vi "DigitalToString.vi"(2 "D3":bool, 3 "D2":bool, 4 "D1":bool) -> (0 "Numeric":dbl, 1 "String":string)   [LabVIEW 2014]
panel:
  out "Led 3":bool
  out "Led 2":bool
  out "Led 1":bool
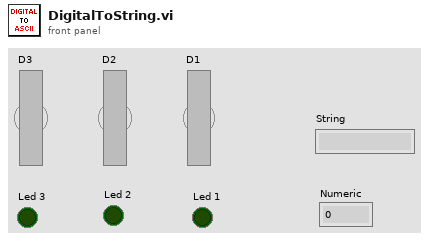
[diagram p1: front panel]
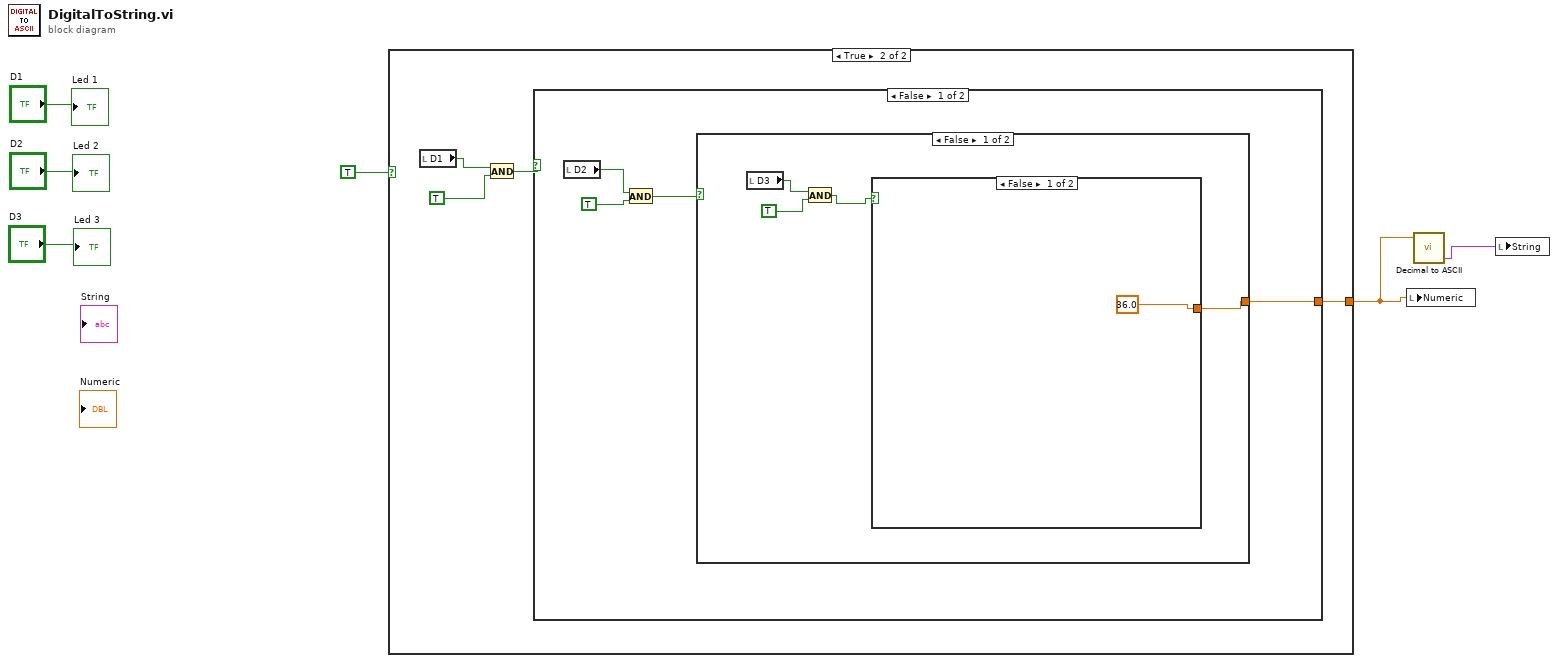
[diagram p0: block diagram]
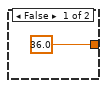
[diagram p2: hidden frame]
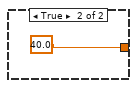
[diagram p3: hidden frame]
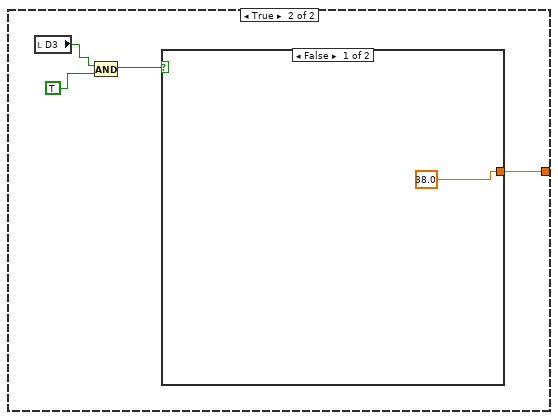
[diagram p4: hidden frame]
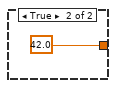
[diagram p5: hidden frame]
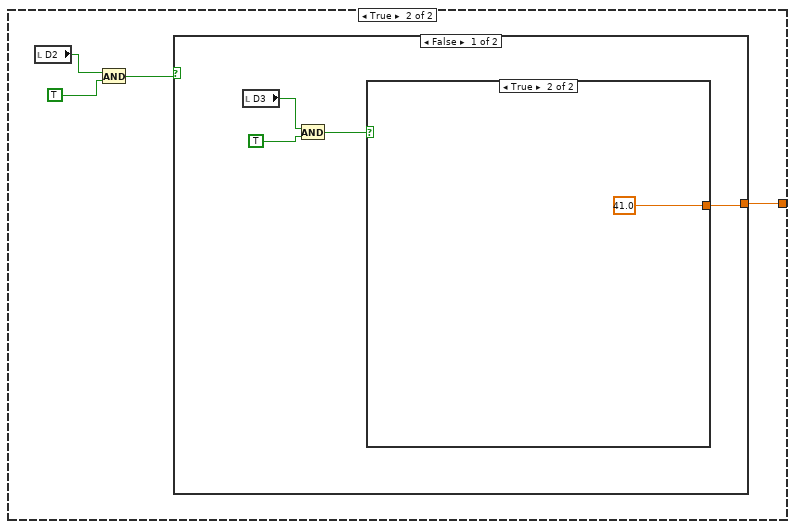
[diagram p6: hidden frame]
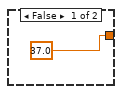
[diagram p7: hidden frame]
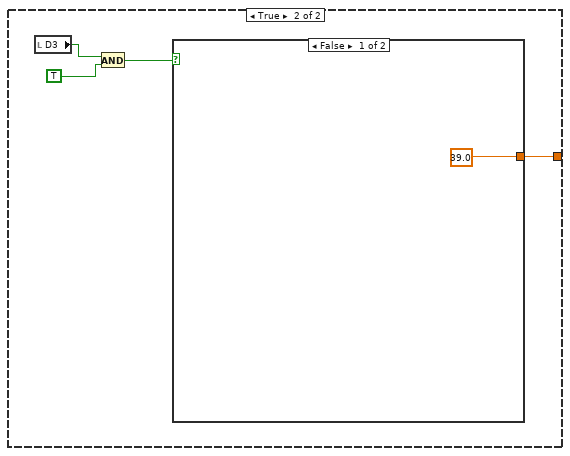
[diagram p8: hidden frame]
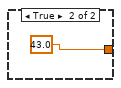
[diagram p9: hidden frame]
diagram:
  n1 = case shown="True" TRUE {
    tunnel: [36.0 ("Numeric") w8] -> w2
    frame False {
    }
    frame True {
      n2 = local read "D1"() -> (w11:bool)
      n3 = And(x=w11, y=TRUE) -> (x .and. y?=w9:bool)
      n4 = case shown="False" w9 {
        tunnel: [w12 w28] -> w8
        frame False {
          n5 = local read "D2"() -> (w14:bool)
          n6 = And(x=w14, y=TRUE) -> (x .and. y?=w13:bool)
          n7 = case shown="False" w13 {
            tunnel: [w16 w22] -> w12
            frame False {
              n8 = local read "D3"() -> (w19:bool)
              n9 = And(x=w19, y=TRUE) -> (x .and. y?=w17:bool)
              n10 = case shown="False" w17 {
                tunnel: [36.0 40.0] -> w16
                frame False {
                }
                frame True {
                }
              }
            }
            frame True {
              n11 = local read "D3"() -> (w25:bool)
              n12 = And(x=w25, y=TRUE) -> (x .and. y?=w23:bool)
              n13 = case shown="False" w23 {
                tunnel: [38.0 42.0] -> w22
                frame False {
                }
                frame True {
                }
              }
            }
          }
        }
        frame True {
          n14 = local read "D2"() -> (w31:bool)
          n15 = And(x=w31, y=TRUE) -> (x .and. y?=w29:bool)
          n16 = case shown="False" w29 {
            tunnel: [w32 w38] -> w28
            frame False {
              n17 = local read "D3"() -> (w35:bool)
              n18 = And(x=w35, y=TRUE) -> (x .and. y?=w33:bool)
              n19 = case shown="True" w33 {
                tunnel: [37.0 41.0] -> w32
                frame False {
                }
                frame True {
                }
              }
            }
            frame True {
              n20 = local read "D3"() -> (w41:bool)
              n21 = And(x=w41, y=TRUE) -> (x .and. y?=w39:bool)
              n22 = case shown="False" w39 {
                tunnel: [39.0 43.0] -> w38
                frame False {
                }
                frame True {
                }
              }
            }
          }
        }
      }
    }
  }
  n23 = local write "Numeric"(w2) -> ()
  n24 = call "Decimal to ASCII.vi"("Decimal Number"=w2) -> ("ASCII Character"=w1:string)  [unwired: 2 in, 2 out]
  n25 = local write "String"(w1) -> ()
  "Led 1" <- "D1"
  "Led 2" <- "D2"
  "Led 3" <- "D3"
